vi "Read Element of STRANS.vi"(8 "error in (no error)":errorcluster, 10 "index":i32, 11 "Referential in":refnum<class "Referential.lvclass">) -> (0 "error out":errorcluster, 2 "Bit":bool, 3 "Referential out":refnum<class "Referential.lvclass">)   [LabVIEW 2019, in "Referential.lvclass"]
uses:
  Referential.lvclass
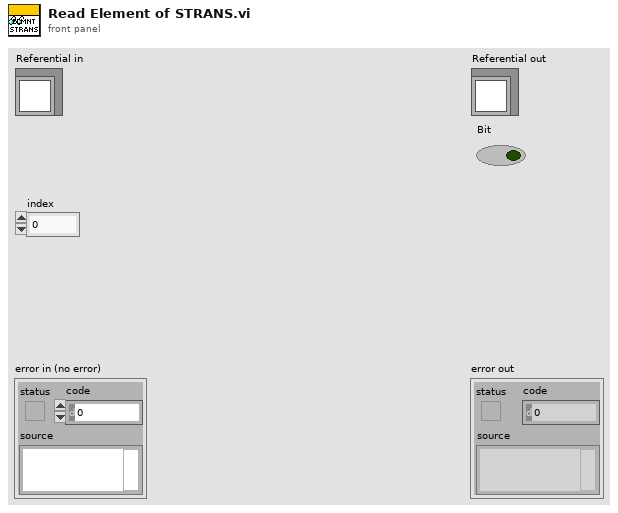
[diagram p1: front panel]
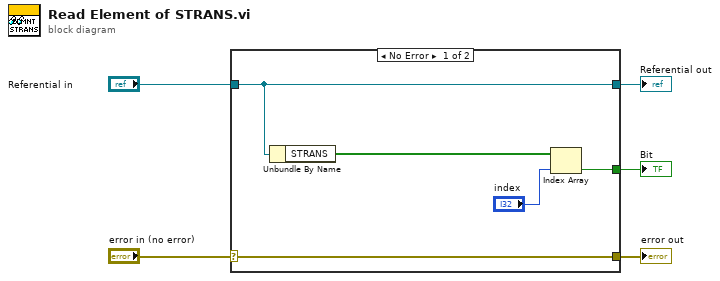
[diagram p0: block diagram]
diagram:
  n1 = case shown="No Error" "error in (no error)" {
    selector: "error in (no error)" -> [w10 w11]
    tunnel: [w10 w11] -> w4
    tunnel: [w9 w12] -> w2
    tunnel: "Referential in" -> [w9 w12]
    tunnel: [w6 _] -> w1
    frame No Error {
      n2 = Unbundle By Name(w9) -> ("STRANS"=w8:bool[])
      n3 = Index Array(array=w8, index="index") -> (element=w6:bool)
    }
    frame Error {
    }
  }
  "error out" <- w4
  "Referential out" <- w2
  "Bit" <- w1
